vi "VideoCapture_old.vi"(0 "Output Directory":path=path "C:/Users/dpl/OneDrive - Aberystwyth University/Documents/LabVIEW Data/VideoTest", 1 "BaseFilename":string, 3 "error in (no error)":errorcluster, 4 "Path to FFMPEG":path=path "C:/Users/dpl/Downloads/ffmpeg-master-latest-win64-gpl/ffmpeg-master-latest-win64-gpl/bin/ffmpeg.exe", 5 "Duration (s)":dbl=1.0 min=0.0 max=100.0) -> (10 "error out":errorcluster)   [LabVIEW 2024]
doc: "Calls FFMPEG to capture and record a video clip.\nVideo clip is stored in sub-directory VIDEOS from Output directory\n\nFilename derived from Cycle count and nominal temperature (TNOM)\nVideo stampedwith timecode, cycle count and nominal temperature"
uses:
  <userlib>/_OpenG.lib/string/string.llb/openg_string.lvlib
panel:
  out "return code":i32
  out "command string":string
  out "standard error":string
  out "standard output":string
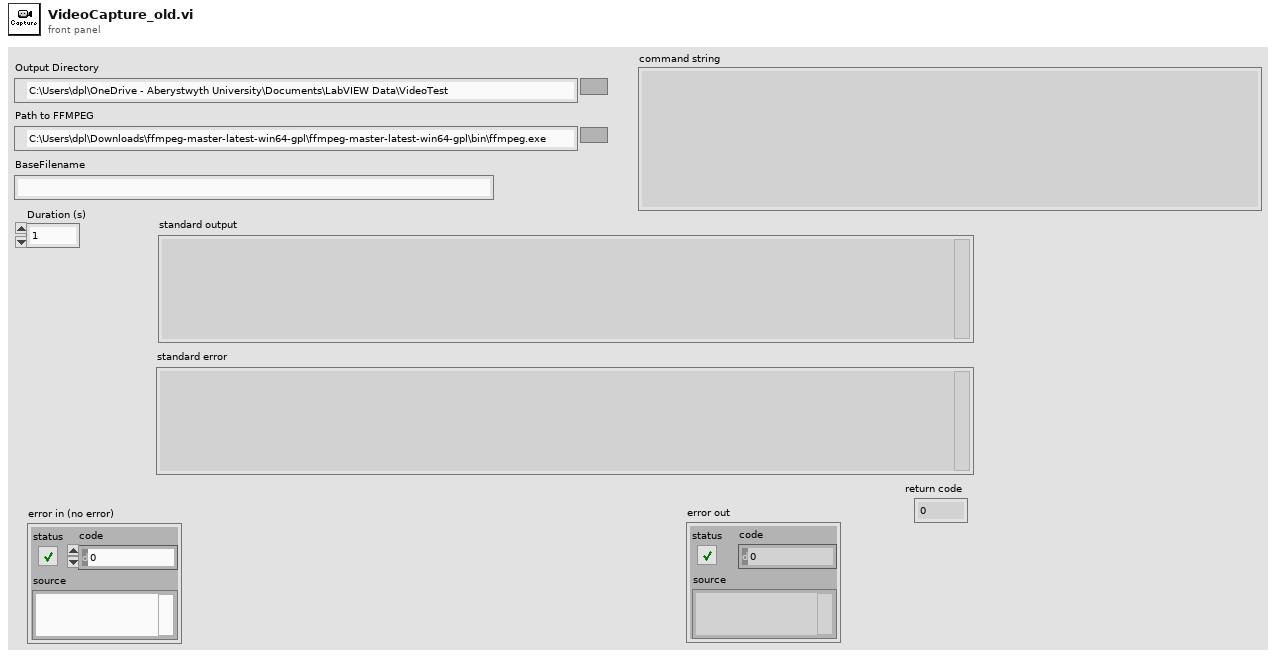
[diagram p1: front panel]
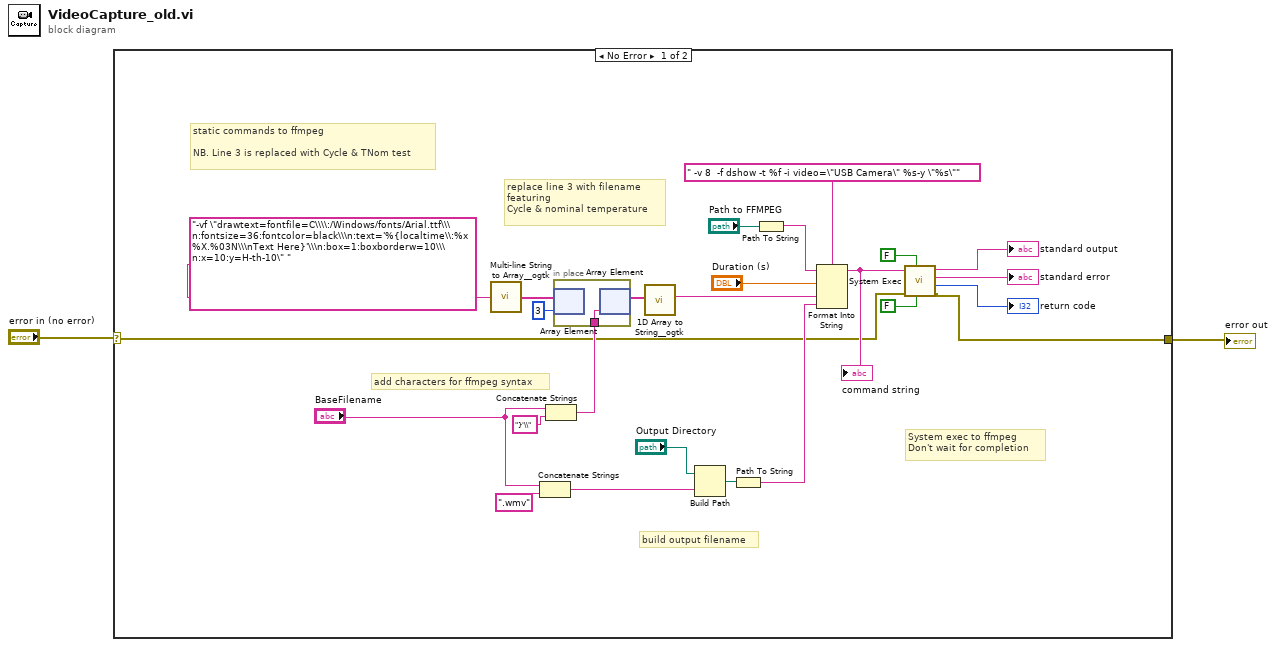
[diagram p0: block diagram]
diagram:
  n1 = case shown="No Error" "error in (no error)" {
    selector: "error in (no error)" -> [w3 w29]
    tunnel: [w4 w29] -> w1
    frame No Error {
      # "add characters for ffmpeg syntax"
      # "build output filename"
      # "System exec to ffmpeg\nDon't wait for completion"
      # "replace line 3 with filename \nfeaturing \nCycle & nominal temperature"
      # "static commands to ffmpeg\n\nNB. Line 3 is replaced with Cycle & TNom test"
      n2 = call <userlib>:"Multi-line String to Array__ogtk.vi"("string"="-vf \"drawtext=fontfile=C\\\\:/Windows/fonts/Arial.ttf\\\n:fontsize=36:fontcolor=black\\\n:text='%{localtime\\:%x %X.%03N\\\nText Here}'\\\n:box=1:boxborderw=10\\\n:x=10:y=H-th-10\" ") -> ("lines"=w14:string[])
      n3 = Concatenate Strings("BaseFilename", ".wmv" ("string")) -> (w7:string)
      n4 = Concatenate Strings("BaseFilename", "}'\\" ("string")) -> (w9:string)
      n5 = in-place {
        in-place-border: w9 -> [w28]
        n6 = in-place-array #1(w14, 3) -> ()  [unwired: 1 out]
        n7 = in-place-array #1(w28) -> (w12:string[])  [unwired: 1 out]
      }
      n8 = call <userlib>:"1D Array to String__ogtk.vi"("Array of Strings"=w12) -> ("delimited string"=w11:string)  [unwired: 10 in]
      n9 = Build Path(base path="Output Directory", name or relative path=w7) -> (appended path=w24:path)
      n10 = Path To String(path=w24) -> (string=w16:string)
      n11 = Path To String(path="Path to FFMPEG") -> (string=w19:string)
      n12 = Format Into String(format string=" -v 8  -f dshow -t %f -i video=\"USB Camera\" %s-y \"%s\"", initial string=w19, "Duration (s)", w11, w16) -> (resulting string=w17:string)  [unwired: 1 in, 1 out]
      "command string" <- w17
      n13 = call <vilib>:"System Exec.vi"("run minimized? (F)"=FALSE, "wait until completion? (T)"=FALSE, "error in (no error)"=w3, "command line"=w17) -> ("error out"=w4:errorcluster, "return code"=→"return code":i32, "standard error"=→"standard error":string, "standard output"=→"standard output":string)  [unwired: 4 in]
    }
    frame Error {
    }
  }
  "error out" <- w1
